vi "Fill FN - Post-Hydrate Wait (SubVI).vi"(0 "Signals IN":T2={"Dispense"=FALSE, "Fill"=FALSE, "Spray"=FALSE, "Drain"=TRUE, "Complete"=FALSE, "Fill Error"=FALSE, "Dispense Error"=FALSE, "Fill Timeout"=FALSE, "Dispense Timeout"=FALSE}, 1 "Values IN":T1 {"Drain Time (s)" format="%.2f"; "Drain Rate (g/sec)" format="%.2f"}, 2 "Measured Mass (g)":dbl(knob) scale=0.0..1000.0, 3 "Settings":T3={"ON Settings"={"Enable Dynamic Setpoint?"=TRUE, "Enable Dynamic Dispense Time?"=TRUE, "Enable Drain Rate Functions"=TRUE, "Dispense Sample Time (s)"=0.5, "Dispense Slope Ave"=0, "ON Timeout (sec)"=600.0, "1st Setpoint (% of Target)"=0.0, "2nd Setpoint (% of Target)"=0.0, "3rd Setpoint (% of Target)"=0.0, "Measure Dispense Delay (sec)"=0.0, "Settle Slope Sample Time (s)"=0.0}, "OFF Settings"={"Drain Sample Time (s)"=0.5, "Drain Rate Ave Size"=5, "Drain Rate Limits (± g/sec)"=10.0, "Level Slope Range (± g/sec)"=0.25, "OFF Timeout (sec)"=0.0, "Near SP Slope Level (± g/sec)"=0.01, "Near Setpoint Threshold (%)"=95.0}, "Overshoot Settings"={"Time Limit (s)"=60.0, "Container MAX (g)"=1500.0, "Max FILL Slope (+/- g/sec)"=10.0, "% Overshot to Enable (>)"=0.25}, "FILL Timeout (s)"=300.0, "Full Settle Time (s)"=20.0, "Pre-Hydrate \nSpray Time (s)"=10.0, "Pre-Hydrate \nWait Time (s)"=30.0}, 5 "Fill Case Change?":bool) -> (14 "Signals OUT":T2, 15 "Values OUT":T1, 19 "Case Complete":bool)   [LabVIEW 2012]
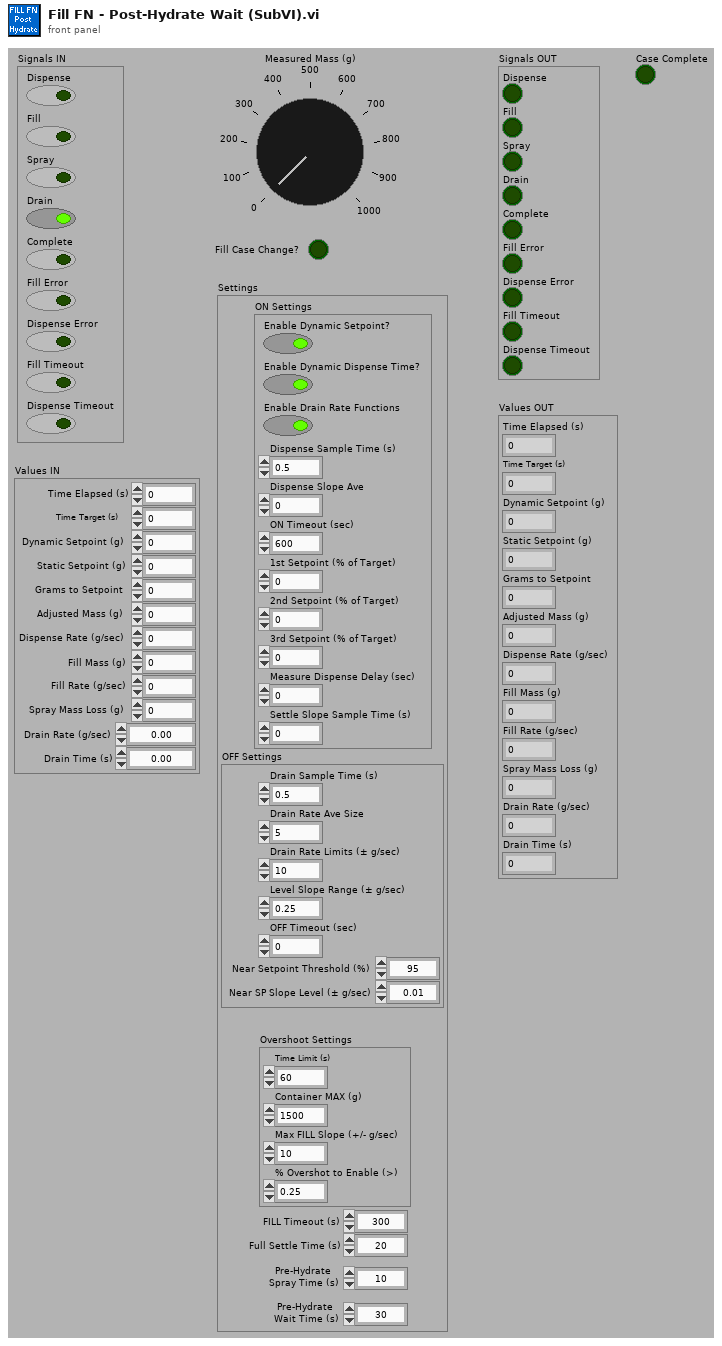
[diagram p1: front panel]
types:
  T1 = cluster{"Time Elapsed (s)":dbl, "Time Target (s)":dbl, "Dynamic Setpoint (g)":dbl, "Static Setpoint (g)":dbl, "Grams to Setpoint":dbl, "Adjusted Mass (g)":dbl, "Dispense Rate (g/sec)":dbl, "Fill Mass (g)":dbl, "Fill Rate (g/sec)":dbl, "Spray Mass Loss (g)":dbl, "Drain Rate (g/sec)":dbl, "Drain Time (s)":dbl}
  T2 = cluster{"Dispense":bool, "Fill":bool, "Spray":bool, "Drain":bool, "Complete":bool, "Fill Error":bool, "Dispense Error":bool, "Fill Timeout":bool, "Dispense Timeout":bool}
  T3 = cluster{"ON Settings":cluster{"Enable Dynamic Setpoint?":bool, "Enable Dynamic Dispense Time?":bool, "Enable Drain Rate Functions":bool, "Dispense Sample Time (s)":dbl, "Dispense Slope Ave":i32, "ON Timeout (sec)":dbl, "1st Setpoint (% of Target)":dbl, "2nd Setpoint (% of Target)":dbl, "3rd Setpoint (% of Target)":dbl, "Measure Dispense Delay (sec)":dbl, "Settle Slope Sample Time (s)":dbl}, "OFF Settings":cluster{"Drain Sample Time (s)":dbl, "Drain Rate Ave Size":i32, "Drain Rate Limits (± g/sec)":dbl, "Level Slope Range (± g/sec)":dbl, "OFF Timeout (sec)":dbl, "Near SP Slope Level (± g/sec)":dbl, "Near Setpoint Threshold (%)":dbl}, "Overshoot Settings":cluster{"Time Limit (s)":dbl, "Container MAX (g)":dbl, "Max FILL Slope (+/- g/sec)":dbl, "% Overshot to Enable (>)":dbl}, "FILL Timeout (s)":dbl, "Full Settle Time (s)":dbl, "Pre-Hydrate \nSpray Time (s)":dbl, "Pre-Hydrate \nWait Time (s)":dbl}
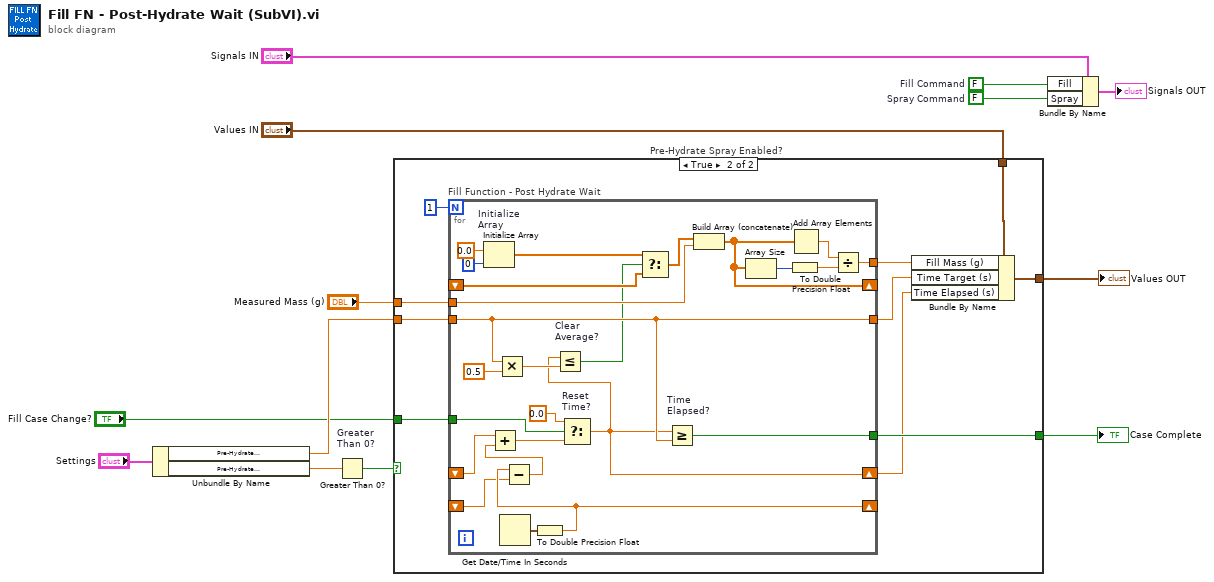
[diagram p0: block diagram]
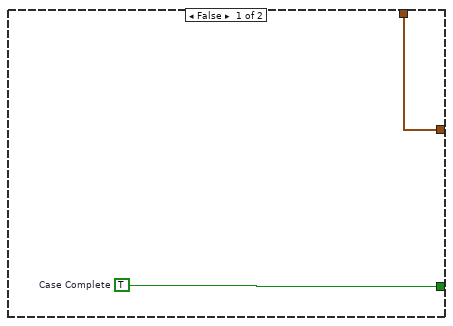
[diagram p2: hidden frame]
diagram:
  w13 = FALSE  # Spray Command
  w6 = FALSE  # Fill Command
  n1 = Unbundle By Name("Settings") -> ("Pre-Hydrate \nWait Time (s)"=w12:dbl, "Pre-Hydrate \nSpray Time (s)"=w2:dbl)
  n2 = Greater Than 0? "Greater\nThan 0?"(x=w2) -> (x > 0?=w3:bool)
  n3 = case "Pre-Hydrate Spray Enabled?" shown="True" w3 {
    tunnel: w12 -> [_ w24]
    tunnel: "Fill Case Change?" -> [_ w22]
    tunnel: "Measured Mass (g)" -> [_ w23]
    tunnel: [w15 w21] -> w9
    tunnel: "Values IN" -> [w15 w20]
    tunnel: [w14 w18] -> w11
    frame False {
      w14 = TRUE  # Case Complete
    }
    frame True {
      n4 = for "Fill Function - Post Hydrate Wait" {
        N: 1 -> [_]
        shift-right: [w49] -> _
        shift-left: _ -> [w48]
        shift-right: [w28] -> w16
        shift-left: _ -> [w46]
        tunnel: w23 -> [w34]
        tunnel: [w33] -> w19
        shift-right: [w41] -> _
        shift-left: _ -> [w35]
        tunnel: [w30] -> w17
        tunnel: [w32] -> w18
        tunnel: w24 -> [w30]
        tunnel: w22 -> [w27]
        n5 = Initialize Array "Initialize\nArray"(0.0 ("Measured Mass (g)"), 0 ("dimension size")) -> (w37:dbl[])
        n6 = Multiply(x=w30, y=0.5) -> (x*y=w29:dbl)
        n7 = Get Date/Time In Seconds() -> (seconds since 1Jan1904=w50:timestamp)
        n8 = To Double Precision Float(number=w50) -> (double precision float=w49:dbl)
        n9 = Subtract(x=w49, y=w48) -> (x-y=w45:dbl)
        n10 = Add(x=w46, y=w45) -> (x+y=w47:dbl)
        n11 = Select "Reset\nTime?"(t=0.0, s=w27, f=w47) -> (s? t:f=w28:dbl)
        n12 = Less Or Equal? "Clear \nAverage?"(x=w28, y=w29) -> (x <= y?=w26:bool)
        n13 = Select(t=w37, s=w26, f=w35) -> (s? t:f=w36:dbl[])
        n14 = Greater Or Equal? "Time\nElapsed?"(x=w28, y=w30) -> (x >= y?=w32:bool)
        n15 = Build Array (concatenate)(w36, w34) -> (w41:dbl[])
        n16 = Array Size(array=w41) -> (size(s)=w39:i32)
        n17 = To Double Precision Float(number=w39) -> (double precision float=w38:dbl)
        n18 = Add Array Elements(numeric array=w41) -> (sum=w40:dbl)
        n19 = Divide(x=w40, y=w38) -> (x/y=w33:dbl)
      }
      n20 = Bundle By Name(cluster=w20, "Fill Mass (g)"=w19, "Time Target (s)"=w17, "Time Elapsed (s)"=w16) -> (w21:T1)
    }
  }
  "Case Complete" <- w11
  "Values OUT" <- w9
  n21 = Bundle By Name(cluster="Signals IN", "Fill"=w6, "Spray"=w13) -> (→"Signals OUT":T2)
